vi "Update JSON.vi"(8 "error in (no error)":errorcluster, 9 "Value":variant, 10 "key":string="data", 11 "JSON in":string) -> (0 "error out":errorcluster, 3 "JSON out":string)   [LabVIEW 2019, in "Shared.lvlib"]
uses:
  Shared.lvlib
  <userlib>/_OpenG.lib/lvdata/lvdata.llb/Type Descriptor Enumeration__ogtk.ctl
  <vilib>/addons/_JKI.lib/Serialization/JSON/JKI JSON Serialization.lvlib
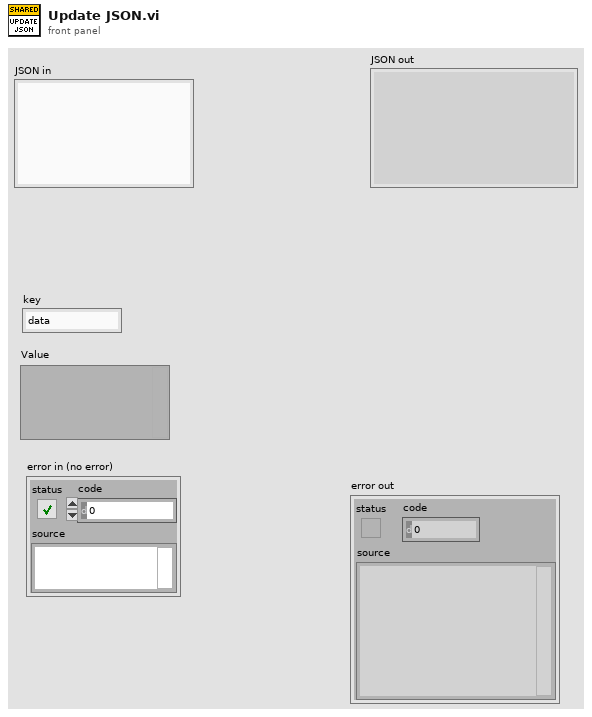
[diagram p1: front panel]
types:
  T1 = typedef "Type Descriptor Enumeration__ogtk.ctl" = enum8{"<Null>", "I8", "I16", "I32", "I64", "U8", "U16", "U32", "U64", "SGL", "DBL", "EXT", "CSG", "CDB", "CXT", "0x0F", "0x10", "0x11", "0x12", "0x13", "0x14", "Enum U8", "Enum U16", "Enum U32", "Enum U64", "SGL PQ", "DBL PQ", "EXT PQ", "CSG PQ", "CDB PQ", "CXT PQ", "0x1F", "0x20", "Boolean", "0x22", "0x23", "0x24", "0x25", "0x26", "0x27", "0x28", "0x29", "0x2A", "0x2B", "0x2C", "0x2D", "0x2E", "0x2F", "String", "0x31", "Path", "Pict", "0x34", "0x35", "0x36", "DAQ", "0x38", "0x39", "0x3A", "0x3B", "0x3C", "0x3D", "0x3E", "0x3F", "Array", "0x41", "0x42", "0x43", "0x44", "0x45", "0x46", "0x47", "0x48", "0x49", "0x4A", "0x4B", "0x4C", "0x4D", "0x4E", "0x4F", "Cluster", "0x51", "0x52", "Variant", "Waveform", "0x55", "0x56", "0x57", "0x58", "0x59", "0x5A", "0x5B", "0x5C", "0x5D", "0x5E", "0x5F", "0x60", "0x61", "0x62", "0x63", "0x64", "0x65", "0x66", "0x67", "0x68", "0x69", "0x6A", "0x6B", "0x6C", "0x6D", "0x6E", "0x6F", "Refnum"}
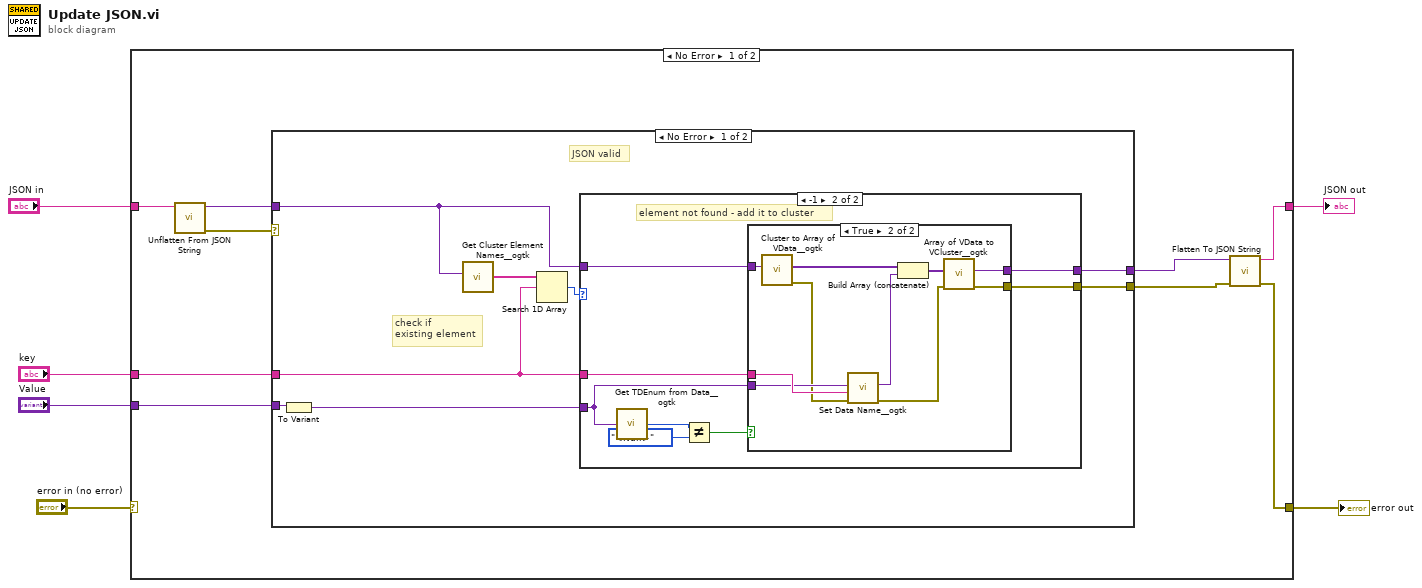
[diagram p0: block diagram]
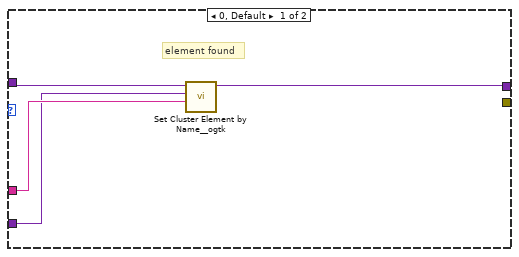
[diagram p2: hidden frame]
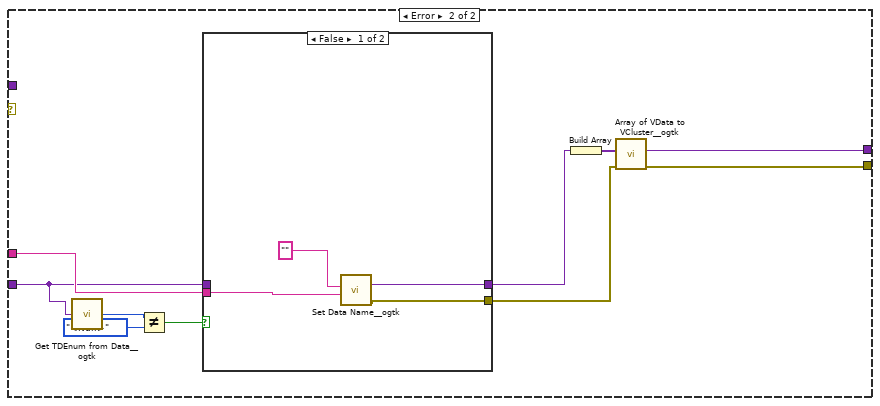
[diagram p4: hidden frame]
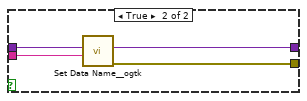
[diagram p5: hidden frame]
diagram:
  n1 = case shown="No Error" "error in (no error)" {
    selector: "error in (no error)" -> [_ w66]
    tunnel: "JSON in" -> [w15 w65]
    tunnel: [w14 w65] -> w5
    tunnel: "key" -> [w12 _]
    tunnel: [w9 w66] -> w3
    tunnel: "Value" -> [w8 _]
    frame No Error {
      n2 = call <vilib>:"Unflatten From JSON String.vi"("JSON String"=w15) -> ("error out"=w7:errorcluster, "Variant"=w13:variant)  [unwired: 9 in]
      n3 = case shown="No Error" w7 {
        tunnel: w13 -> [w21 _]
        tunnel: w12 -> [w20 w56]
        tunnel: [w19 w47] -> w11
        tunnel: [w18 w48] -> w10
        tunnel: w8 -> [w16 w53]
        frame No Error {
          # "check if\nexisting element"
          # "JSON valid"
          n4 = To Variant(anything=w16) -> (Variant=w17:variant)
          n5 = call <userlib>:"Get Cluster Element Names__ogtk.vi"("Cluster"=w21) -> ("Element Names"=w23:string[])  [unwired: 9 in, 1 out]
          n6 = Search 1D Array(1D array=w23, element=w20) -> (index of element=w22:i32)  [unwired: 1 in]
          n7 = case shown="-1" w22 {
            tunnel: w21 -> [w27 w34]
            tunnel: w20 -> [w26 w35]
            tunnel: w17 -> [w25 w32]
            tunnel: [w24 w33] -> w19
            tunnel: [_ w31] -> w18
            frame 0, Default {
              # "element found"
              n8 = call <userlib>:"Set Cluster Element by Name__ogtk.vi"("Element Name (\"\": New Element Data Name)"=w26, "New Element Value"=w25, "Cluster"=w27) -> ("VCluster out"=w24:variant)  [unwired: 6 in, 2 out]
            }
            frame -1 {
              # "element not found - add it to cluster"
              n9 = call <userlib>:"Get TDEnum from Data__ogtk.vi"("Data"=w32) -> ("Type Descriptor Enumeration"=w30:T1)  [unwired: 4 in]
              n10 = Not Equal?(x=w30, y=Type_Descriptor_Enumeration__ogtk."<Null>") -> (x != y?=w28:bool)
              n11 = case shown="True" w28 {
                tunnel: w35 -> [_ w46]
                tunnel: w34 -> [w36 w44]
                tunnel: [w36 w42] -> w33
                tunnel: w32 -> [_ w41]
                tunnel: [_ w38] -> w31
                frame False {
                }
                frame True {
                  n12 = call <userlib>:"Cluster to Array of VData__ogtk.vi"("Cluster"=w44) -> ("error out"=w40:errorcluster, "Array of VData"=w37:variant[])  [unwired: 9 in]
                  n13 = call <userlib>:"Set Data Name__ogtk.vi"("error in (no error)"=w40, "Data Name"=w46, "Data"=w41) -> ("error out"=w39:errorcluster, "Renamed Data"=w43:variant)  [unwired: 7 in]
                  n14 = Build Array (concatenate)(w37, w43) -> (w45:variant[])
                  n15 = call <userlib>:"Array of VData to VCluster__ogtk.vi"("error in (no error)"=w39, "Array"=w45) -> ("error out"=w38:errorcluster, "VCluster"=w42:variant)  [unwired: 8 in]
                }
              }
            }
          }
        }
        frame Error {
          n16 = call <userlib>:"Get TDEnum from Data__ogtk.vi"("Data"=w53) -> ("Type Descriptor Enumeration"=w55:T1)  [unwired: 4 in]
          n17 = Not Equal?(x=w55, y=Type_Descriptor_Enumeration__ogtk."<Null>") -> (x != y?=w52:bool)
          n18 = case shown="False" w52 {
            tunnel: w56 -> [w59 w64]
            tunnel: w53 -> [_ w63]
            tunnel: [w58 w62] -> w50
            tunnel: [w57 w61] -> w49
            frame False {
              n19 = call <userlib>:"Set Data Name__ogtk.vi"("Data Name"=w59, "Data"="") -> ("error out"=w57:errorcluster, "Renamed Data"=w58:variant)  [unwired: 8 in]
            }
            frame True {
              n20 = call <userlib>:"Set Data Name__ogtk.vi"("Data Name"=w64, "Data"=w63) -> ("error out"=w61:errorcluster, "Renamed Data"=w62:variant)  [unwired: 8 in]
            }
          }
          n21 = Build Array(w50) -> (w51:variant[])
          n22 = call <userlib>:"Array of VData to VCluster__ogtk.vi"("error in (no error)"=w49, "Array"=w51) -> ("error out"=w48:errorcluster, "VCluster"=w47:variant)  [unwired: 8 in]
        }
      }
      n23 = call <vilib>:"Flatten To JSON String.vi"("error in (no error)"=w10, "Variant"=w11) -> ("error out"=w9:errorcluster, "JSON String"=w14:string)  [unwired: 8 in]
    }
    frame Error {
    }
  }
  "JSON out" <- w5
  "error out" <- w3
